vi "Kalibrierdaten.vi"() -> ()   [LabVIEW 2020, in "ABB-EL3000.lvlib" / "Allgemeine VI.lvlib"]
uses:
  Allgemeine VI.lvlib
  Visualisierungs Elemente/Button.ctl
  Visualisierungs Elemente/Zahlen-Ausgabefeld.ctl
  Visualisierungs Elemente/Zahlen-Eingabefeld.ctl
  Auto Kalibrieren/Aktionen FGV AutoKAL Daten.ctl
  FGV Uras26 Aktion.ctl
  CAL-Daten Toleranz.ctl
  Aktionen Cal Daten speichern.ctl
  PMA/Kalibrieren/Kalibrieren.lvlib
  Allgemein/allgemeine Sub-VIs.lvlib
  Auto Kalibrieren/Auto Kalibrieren.lvlib
  FID/FID Kalibrierung/FID Kalibrierung.lvlib
panel:
  out "THC End 3":T1 format="%.4f"
  out "THC End 2":T1 format="%.4f"
  in  "O2 Zeit-E":T2 format="%#_5g"
  in  "O2 Zeit-0":T2 format="%#_5g"
  in  "O2 0-Grund.":T2 format="%#_5g"
  in  "O2 0-KAL":T2 format="%#_5g"
  in  "O2 E-Grund.":T2 format="%#_5g"
  in  "O2 E-KAL":T2 format="%#_5g"
  out "O2 Null":T1 format="%.4f"
  out "O2 End":T1 format="%.4f"
  in  "THC Zeit-E":T2 format="%#_5g"
  in  "THC Zeit-0":T2 format="%#_5g"
  in  "THC 0-Grund.":T2 format="%#_5g"
  in  "THC 0-KAL":T2 format="%#_5g"
  out "THC Null":T1 format="%.4f"
  in  "THC E-Grund.":T2 format="%#_5g"
  in  "THC E-KAL":T2 format="%#_5g"
  out "THC End1":T1 format="%.4f"
  in  "CO2 hi Zeit-E":T2 format="%#_5g"
  in  "CO2 hi 0-Grund.":T2 format="%#_5g"
  in  "CO2 hi 0-KAL":T2 format="%#_5g"
  in  "CO2 hi E-Grund.":T2 format="%#_5g"
  in  "CO2 hi E-KAL":T2 format="%#_5g"
  out "CO2 hi Null":T1 format="%.4f"
  out "CO2 hi End1":T1 format="%.4f"
  in  "CO2 hi Zeit-0":T2 format="%#_5g"
  in  "CO2 lo Zeit-E":T2 format="%#_5g"
  in  "CO2 lo 0-Grund.":T2 format="%#_5g"
  in  "CO2 lo 0-KAL":T2 format="%#_5g"
  out "CO2 lo Null":T1 format="%.4f"
  in  "CO2 lo E-Grund.":T2 format="%#_5g"
  in  "CO2 lo E-KAL":T2 format="%#_5g"
  out "CO2 lo End2":T1 format="%.4f"
  out "CO2 lo End1":T1 format="%.4f"
  in  "CO2 lo Zeit-0":T2 format="%#_5g"
  in  "CH4 Zeit-E":T2 format="%#_5g"
  in  "CH4 Zeit-0":T2 format="%#_5g"
  in  "CH4 0-Grund.":T2 format="%#_5g"
  in  "CH4 0-KAL":T2 format="%#_5g"
  in  "CH4 E-Grund.":T2 format="%#_5g"
  in  "CH4 E-KAL":T2 format="%#_5g"
  out "CH4 Null":T1 format="%.4f"
  out "CH4 End1":T1 format="%.4f"
  in  "CO lo Zeit-E":T2 format="%#_5g"
  in  "CO lo Zeit-0":T2 format="%#_5g"
  in  "CO lo 0-Grund.":T2 format="%#_5g"
  in  "CO lo 0-KAL":T2 format="%#_5g"
  out "CO lo Null":T1 format="%.4f"
  out "CO lo End3":T1 format="%.4f"
  in  "CO lo E-Grund.":T2 format="%#_5g"
  in  "CO lo E-KAL":T2 format="%#_5g"
  out "CO lo End2":T1 format="%.4f"
  out "CO lo End1":T1 format="%.4f"
  in  "speichern":T3
  in  "ABBRECHEN":T3
  # "0-Punkt"
  # "End-Punkt"
  # "0-Punkt Toleranz [abs]"
  # "End-Punkt Toleranz [%]"
  # "Aufschaltzeit Auto-KAL [sec]"
  # "letzte\nKalibrierung"
  # "Grund-\nkalibrierung"
  # "letzte\nKalibrierung"
  # "Grund-\nkalibrierung"
  # "0-Punkt"
  # "End-Punkt"
  # "MB 1"
  # "MB 2"
  # "MB 3"
  # "THC:"
  # "O2:"
  # "reserve:"
  # "CO2 lo:"
  # "CH4:"
  # "CO lo:"
  # "Kalibrierdaten"
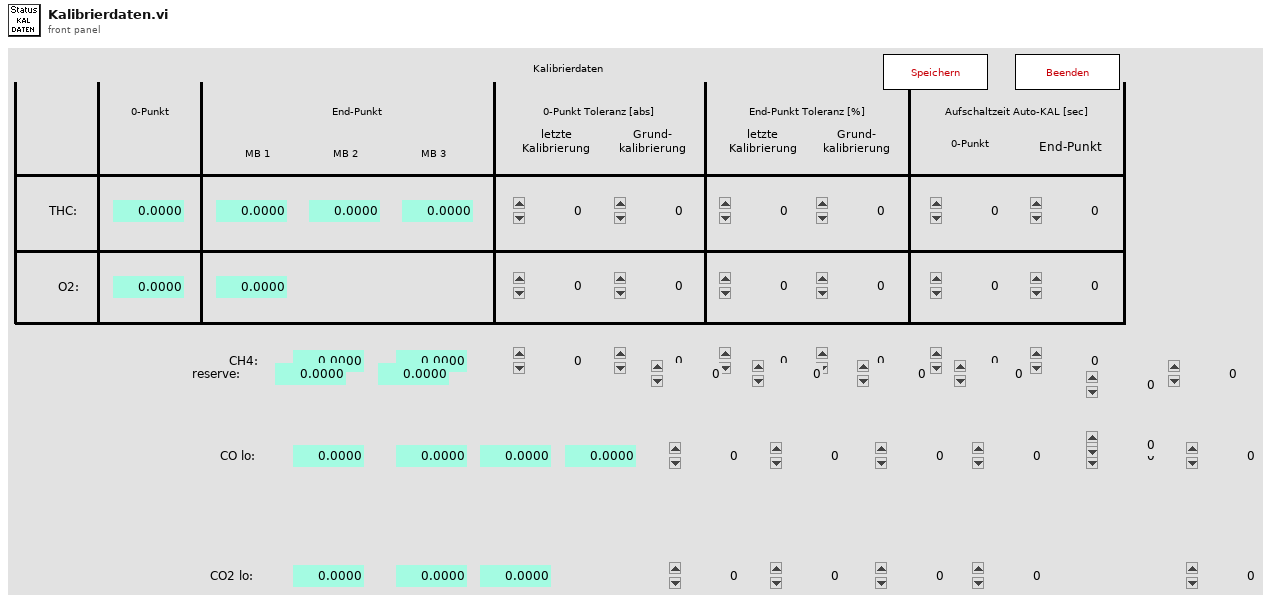
[diagram p1: front panel]
types:
  T1 = typedef "Zahlen-Ausgabefeld.ctl" = sgl
  T2 = typedef "Zahlen-Eingabefeld.ctl" = sgl
  T3 = typedef "Button.ctl" = bool
  T4 = typedef "ABB-EL3000.lvlib/Allgemeine VI.lvlib/FGV Uras26 Aktion.ctl" = enum16{"lesen", "CAL-Daten laden", "Messen", "Kalibrieren vorbereiten", "Kalibrieren", "CAL-Daten speichern", "Toleranz schreiben", "CAL-Daten kopieren"}
  T5 = typedef "Auto Kalibrieren.lvlib/Aktionen FGV AutoKAL Daten.ctl" = enum16{"lesen", "laden", "speichern", "Aufschaltzeit"}
  T6 = typedef "ABB-EL3000.lvlib/Allgemeine VI.lvlib/CAL-Daten Toleranz.ctl" = cluster{"CO lo 0-KAL":sgl, "CO lo 0-Grund":sgl, "CO lo E-KAL":sgl, "CO lo E-Grund":sgl, "CO hi 0-KAL":sgl, "CO hi 0-Grund":sgl, "CO hi E-KAL":sgl, "CO hi E-Grund":sgl, "CH4 0-KAL":sgl, "CH4 0-Grund":sgl, "CH4 E-KAL":sgl, "CH4 E-Grund":sgl, "THC 0-KAL":sgl, "THC 0-Grund":sgl, "THC E-KAL":sgl, "THC E-Grund":sgl, "NMHC 0-KAL":sgl, "NMHC 0-Grund":sgl, "NMHC E-KAL":sgl, "NMHC E-Grund":sgl, "O2 0-KAL":sgl, "O2 0-Grund":sgl, "O2 E-KAL":sgl, "O2 E-Grund":sgl}
  T7 = typedef "Auto Kalibrieren.lvlib/Auschaltzeiten Null Endpunktgase.ctl" = cluster{"CO lo 0":sgl, "CO lo E":sgl, "CO hi 0":sgl, "CO hi E":sgl, "CO2 lo 0":sgl, "CO2 lo E":sgl, "CH4 0":sgl, "CH4 E":sgl, "THC 0":sgl, "THC E":sgl, "O2 0":sgl, "O2 E":sgl}
  T8 = typedef "ABB-EL3000.lvlib/Allgemeine VI.lvlib/Aktionen Cal Daten speichern.ctl" = enum16{"Cal Daten", "Toleranzen", "PMA", "FID", "Cal Daten PMA", "Cal Daten FID"}
  T9 = typedef "ABB-EL3000.lvlib/Allgemeine VI.lvlib/CAL-Daten PMA.ctl" = cluster{"O2 Null":sgl, "O2 Steil":sgl[]}
  T10 = typedef "ABB-EL3000.lvlib/Allgemeine VI.lvlib/CAL-Daten FID.ctl" = cluster{"CH4 Null":sgl, "CH4 Steil":sgl[], "THC Null":sgl, "THC Steil":sgl[], "NMHC Null":sgl, "NMHC Steil":sgl[]}
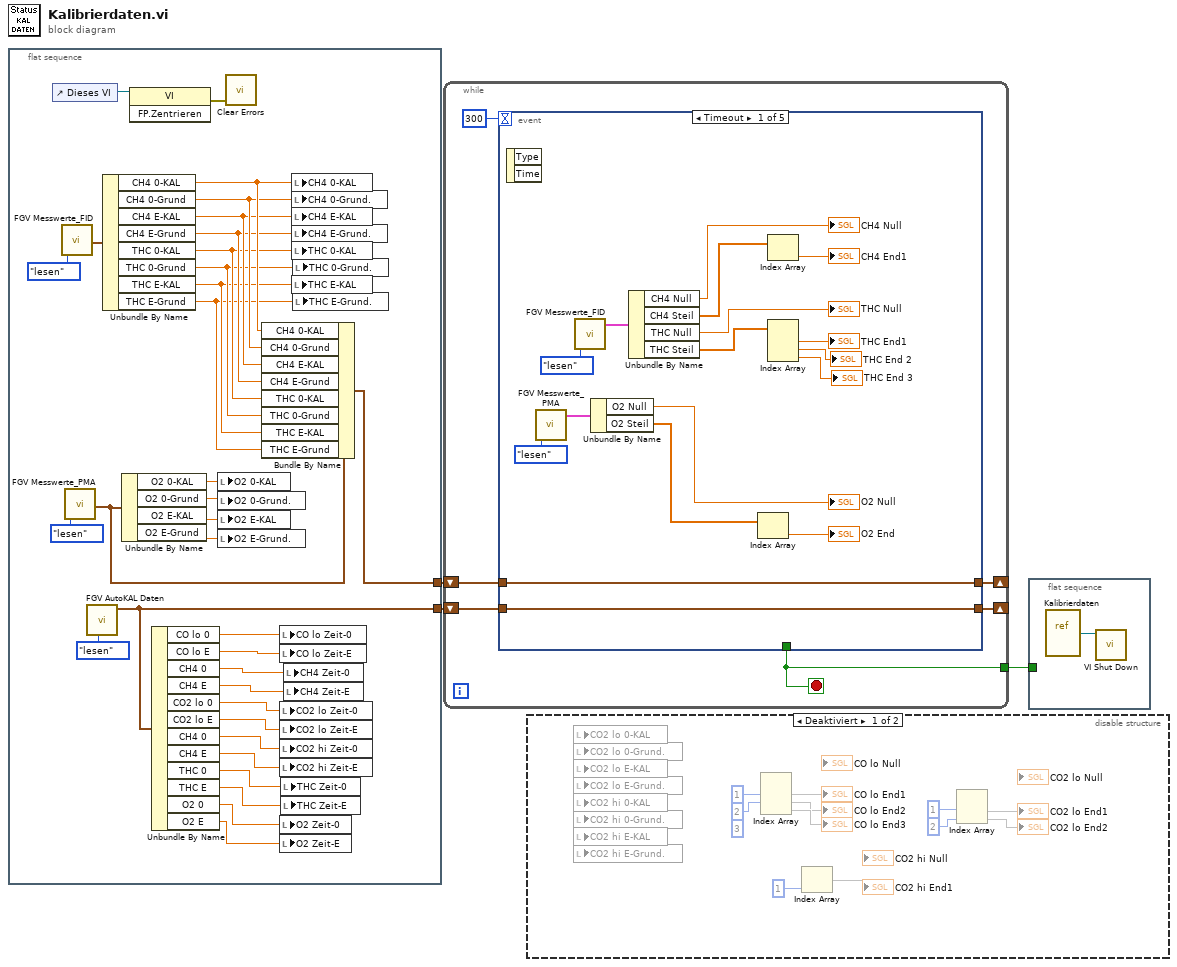
[diagram p0: block diagram]
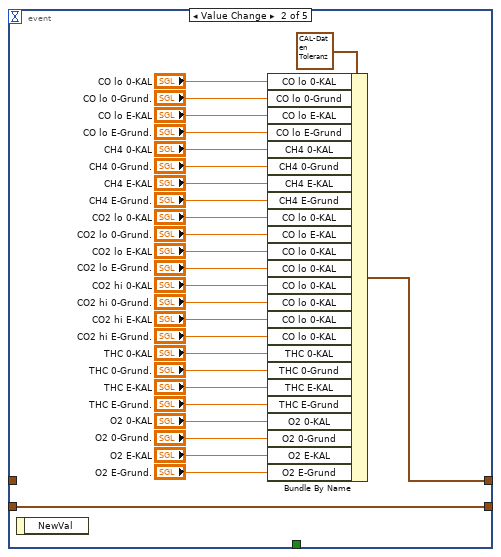
[diagram p3: hidden frame]
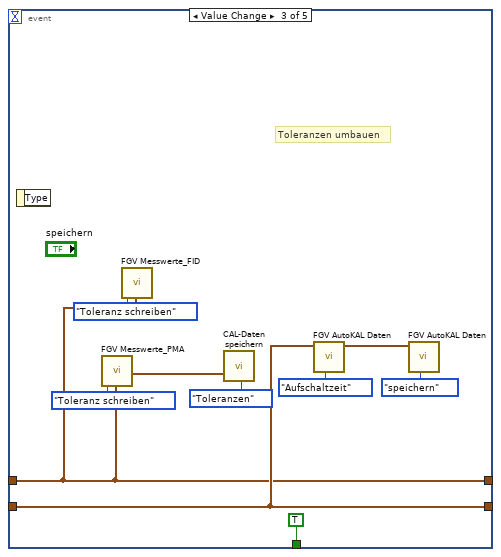
[diagram p4: hidden frame]
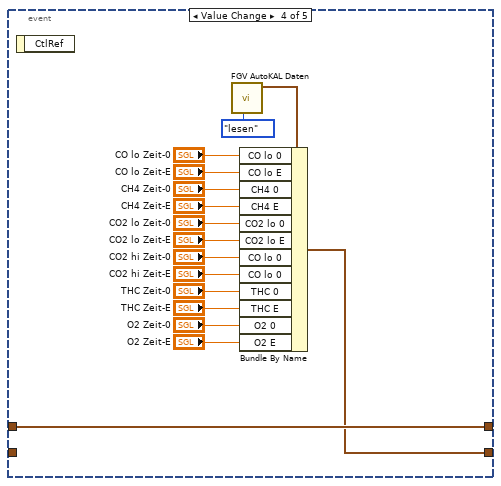
[diagram p5: hidden frame]
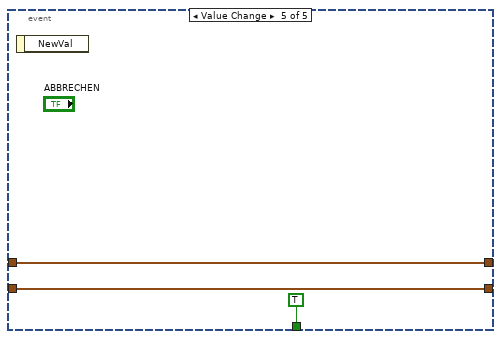
[diagram p6: hidden frame]
diagram:
  n1 = flat-sequence {
    tunnel: [w12] -> w2
    tunnel: [w33] -> w1
    frame #0 {
      n2 = control-ref of="Dieses VI"() -> (w16:refnum<vi>)
      n3 = call "FGV Messwerte_FID.vi"("Aktion"=FGV_Uras26_Aktion."lesen") -> ("CAL-Daten Tolernaz"=w13:T6)  [unwired: 19 in, 7 out]
      n4 = call "FGV Messwerte_PMA.vi"("Aktion"=FGV_Uras26_Aktion."lesen") -> ("CAL-Daten Tolernaz"=w35:T6)  [unwired: 19 in, 7 out]
      n5 = call "FGV AutoKAL Daten.vi"("Aktionen"=Aktionen_FGV_AutoKAL_Daten."lesen") -> ("Aufschaltzeiten"=w33:T7)  [unwired: 10 in]
      n6 = Unbundle By Name(w13) -> ("CH4 0-KAL"=w11:sgl, "CH4 0-Grund"=w10:sgl, "CH4 E-KAL"=w9:sgl, "CH4 E-Grund"=w8:sgl, "THC 0-KAL"=w7:sgl, "THC 0-Grund"=w6:sgl, "THC E-KAL"=w5:sgl, "THC E-Grund"=w4:sgl)
      n7 = Unbundle By Name(w35) -> ("O2 0-KAL"=w20:sgl, "O2 0-Grund"=w19:sgl, "O2 E-KAL"=w18:sgl, "O2 E-Grund"=w17:sgl)
      n8 = invoke class="VI" method="FP.Zentrieren"(reference=w16) -> (error out=w15:errorcluster)  [unwired: 2 in, 2 out]
      n9 = Unbundle By Name(w33) -> ("CO lo 0"=w31:sgl, "CO lo E"=w23:sgl, "CH4 0"=w24:sgl, "CH4 E"=w25:sgl, "CO2 lo 0"=w26:sgl, "CO2 lo E"=w27:sgl, "CH4 0"=w28:sgl, "CH4 E"=w29:sgl, "THC 0"=w30:sgl, "THC E"=w32:sgl, "O2 0"=w22:sgl, "O2 E"=w21:sgl)
      n10 = local write "O2 0-KAL"(w20) -> ()
      n11 = local write "O2 0-Grund."(w19) -> ()
      n12 = local write "O2 E-KAL"(w18) -> ()
      n13 = local write "O2 E-Grund."(w17) -> ()
      n14 = call <vilib>:"Clear Errors.vi"("error in (no error)"=w15) -> ()  [unwired: 5 in, 2 out]
      n15 = Bundle By Name(cluster=w35, "CH4 0-KAL"=w11, "CH4 0-Grund"=w10, "CH4 E-KAL"=w9, "CH4 E-Grund"=w8, "THC 0-KAL"=w7, "THC 0-Grund"=w6, "THC E-KAL"=w5, "THC E-Grund"=w4) -> (w12:T6)
      n16 = local write "CO lo Zeit-0"(w31) -> ()
      n17 = local write "CO lo Zeit-E"(w23) -> ()
      n18 = local write "CO2 lo Zeit-0"(w26) -> ()
      n19 = local write "CO2 lo Zeit-E"(w27) -> ()
      n20 = local write "CO2 hi Zeit-0"(w28) -> ()
      n21 = local write "CO2 hi Zeit-E"(w29) -> ()
      n22 = local write "O2 Zeit-0"(w22) -> ()
      n23 = local write "O2 Zeit-E"(w21) -> ()
      n24 = local write "THC Zeit-0"(w30) -> ()
      n25 = local write "THC Zeit-E"(w32) -> ()
      n26 = local write "CH4 Zeit-0"(w24) -> ()
      n27 = local write "CH4 Zeit-E"(w25) -> ()
      n28 = local write "CH4 0-KAL"(w11) -> ()
      n29 = local write "CH4 0-Grund."(w10) -> ()
      n30 = local write "CH4 E-KAL"(w9) -> ()
      n31 = local write "CH4 E-Grund."(w8) -> ()
      n32 = local write "THC 0-KAL"(w7) -> ()
      n33 = local write "THC E-KAL"(w5) -> ()
      n34 = local write "THC 0-Grund."(w6) -> ()
      n35 = local write "THC E-Grund."(w4) -> ()
    }
  }
  n36 = while {
    tunnel: [w41] -> w3
    shift-right: [w40] -> _
    shift-left: w2 -> [w39]
    shift-right: [w37] -> _
    shift-left: w1 -> [w38]
    stop <- w41 stop-if-true
    n37 = event shown="[0] Timeout" {
      selector: _ -> [_ _ _ _ _]
      dyn-events: _ -> [_ _ _ _ _]
      timeout: 300 -> [_ _ _ _ _]
      tunnel: [_ _ TRUE ("ABBRECHEN") _ TRUE ("ABBRECHEN")] -> w41
      tunnel: [w55 w65 w87 w112 w114] -> w40
      tunnel: w39 -> [w55 _ w87 w112 w114]
      tunnel: w38 -> [w54 w64 w91 _ w113]
      tunnel: [w54 w64 w91 w99 w113] -> w37
      event Timeout {
        n38 = event-data() -> ()  [unwired: 1 in, 2 out]
        n39 = call "FGV Messwerte_PMA.vi"("Aktion"=FGV_Uras26_Aktion."lesen") -> ("CAL-Daten"=w58:T9)  [unwired: 19 in, 7 out]
        n40 = call "FGV Messwerte_FID.vi"("Aktion"=FGV_Uras26_Aktion."lesen") -> ("CAL-Daten"=w49:T10)  [unwired: 19 in, 7 out]
        n41 = Unbundle By Name(w58) -> ("O2 Null"=→"O2 Null":sgl, "O2 Steil"=w52:sgl[])
        n42 = Unbundle By Name(w49) -> ("CH4 Null"=→"CH4 Null":sgl, "CH4 Steil"=w47:sgl[], "THC Null"=→"THC Null":sgl, "THC Steil"=w45:sgl[])
        n43 = Index Array(array=w52) -> (element=→"O2 End":sgl)  [unwired: 1 in]
        n44 = Index Array(array=w47) -> (element=→"CH4 End1":sgl)  [unwired: 1 in]
        n45 = Index Array(array=w45) -> (element #1=→"THC End1":sgl, element #2=→"THC End 2":sgl, element #3=→"THC End 3":sgl)  [unwired: 3 in]
      }
      event Value Change {
        n46 = event-data() -> ()  [unwired: 1 in, 1 out]
        n47 = Bundle By Name(cluster=T6 {"CO lo 0-KAL"=0.0, "CO lo 0-Grund"=0.0, "CO lo E-KAL"=0.0, "CO lo E-Grund"=0.0, "CO hi 0-KAL"=0.0, "CO hi 0-Grund"=0.0, "CO hi E-KAL"=0.0, "CO hi E-Grund"=0.0, "CH4 0-KAL"=0.0, "CH4 0-Grund"=0.0, "CH4 E-KAL"=0.0, "CH4 E-Grund"=0.0, "THC 0-KAL"=0.0, "THC 0-Grund"=0.0, "THC E-KAL"=0.0, "THC E-Grund"=0.0, "NMHC 0-KAL"=0.0, "NMHC 0-Grund"=0.0, "NMHC E-KAL"=0.0, "NMHC E-Grund"=0.0, "O2 0-KAL"=0.0, "O2 0-Grund"=0.0, "O2 E-KAL"=0.0, "O2 E-Grund"=0.0} ("CAL-Daten Tolernaz"), "CO lo 0-KAL"="CO lo 0-KAL", "CO lo 0-Grund"="CO lo 0-Grund.", "CO lo E-KAL"="CO lo E-KAL", "CO lo E-Grund"="CO lo E-Grund.", "CH4 0-KAL"="CH4 0-KAL", "CH4 0-Grund"="CH4 0-Grund.", "CH4 E-KAL"="CH4 E-KAL", "CH4 E-Grund"="CH4 E-Grund.", "CO lo 0-KAL"="CO2 lo 0-KAL", "CO lo E-KAL"="CO2 lo 0-Grund.", "CO lo 0-KAL"="CO2 lo E-KAL", "CO lo 0-KAL"="CO2 lo E-Grund.", "CO lo 0-KAL"="CO2 hi 0-KAL", "CO lo 0-KAL"="CO2 hi 0-Grund.", "CO lo 0-KAL"="CO2 hi E-KAL", "CO lo 0-KAL"="CO2 hi E-Grund.", "THC 0-KAL"="THC 0-KAL", "THC 0-Grund"="THC 0-Grund.", "THC E-KAL"="THC E-KAL", "THC E-Grund"="THC E-Grund.", "O2 0-KAL"="O2 0-KAL", "O2 0-Grund"="O2 0-Grund.", "O2 E-KAL"="O2 E-KAL", "O2 E-Grund"="O2 E-Grund.") -> (w65:T6)
      }
      event Value Change {
        # "Toleranzen umbauen"
        n48 = event-data() -> ()  [unwired: 1 in, 1 out]
        n49 = call "FGV Messwerte_PMA.vi"("Aktion"=FGV_Uras26_Aktion."Toleranz schreiben", "CAL-Daten Tolernaz"=w87) -> ("CAL-Daten Tolernaz"=w93:T6)  [unwired: 18 in, 7 out]
        n50 = call "FGV Messwerte_FID.vi"("Aktion"=FGV_Uras26_Aktion."Toleranz schreiben", "CAL-Daten Tolernaz"=w87) -> ()  [unwired: 18 in, 8 out]
        n51 = call "CAL-Daten speichern.vi"("CAL-Daten Tolernaz"=w93, "Aktionen Kal Daten speichern"=Aktionen_Cal_Daten_speichern."Toleranzen") -> ()  [unwired: 18 in]
        n52 = call "FGV AutoKAL Daten.vi"("Aktionen"=Aktionen_FGV_AutoKAL_Daten."Aufschaltzeit", "Aufschaltzeiten"=w91) -> ("Aufschaltzeiten"=w89:T7)  [unwired: 9 in]
        n53 = call "FGV AutoKAL Daten.vi"("Aktionen"=Aktionen_FGV_AutoKAL_Daten."speichern", "Aufschaltzeiten"=w89) -> ()  [unwired: 9 in, 1 out]
      }
      event Value Change {
        n54 = event-data() -> ()  [unwired: 1 in, 1 out]
        n55 = call "FGV AutoKAL Daten.vi"("Aktionen"=Aktionen_FGV_AutoKAL_Daten."lesen") -> ("Aufschaltzeiten"=w110:T7)  [unwired: 10 in]
        n56 = Bundle By Name(cluster=w110, "CO lo 0"="CO lo Zeit-0", "CO lo E"="CO lo Zeit-E", "CH4 0"="CH4 Zeit-0", "CH4 E"="CH4 Zeit-E", "CO2 lo 0"="CO2 lo Zeit-0", "CO2 lo E"="CO2 lo Zeit-E", "CO lo 0"="CO2 hi Zeit-0", "CO lo 0"="CO2 hi Zeit-E", "THC 0"="THC Zeit-0", "THC E"="THC Zeit-E", "O2 0"="O2 Zeit-0", "O2 E"="O2 Zeit-E") -> (w99:T7)
      }
      event Value Change {
        n57 = event-data() -> ()  [unwired: 1 in, 1 out]
      }
    }
  }
  n58 = disable-structure shown="Deaktiviert" {
    frame Disabled {
      (unwired) 3 ("Index")
      n59 = local read "CO2 lo 0-KAL"() -> ()  [unwired: 1 in]
      n60 = local read "CO2 lo 0-Grund."() -> ()  [unwired: 1 in]
      n61 = local read "CO2 lo E-KAL"() -> ()  [unwired: 1 in]
      n62 = local read "CO2 lo E-Grund."() -> ()  [unwired: 1 in]
      n63 = local read "CO2 hi 0-KAL"() -> ()  [unwired: 1 in]
      n64 = local read "CO2 hi 0-Grund."() -> ()  [unwired: 1 in]
      n65 = local read "CO2 hi E-KAL"() -> ()  [unwired: 1 in]
      n66 = local read "CO2 hi E-Grund."() -> ()  [unwired: 1 in]
      n67 = Index Array(index #1=1 ("Index"), index #2=2 ("Index")) -> (element #1=→"CO lo End1", element #2=→"CO lo End2", element #3=→"CO lo End3")  [unwired: 2 in]
      n68 = Index Array(index=1 ("Index")) -> (element=→"CO2 hi End1")  [unwired: 1 in]
      n69 = Index Array(index #1=1 ("Index"), index #2=2 ("Index")) -> (element #1=→"CO2 lo End1", element #2=→"CO2 lo End2")  [unwired: 1 in]
    }
    frame Enabled {
    }
  }
  n70 = flat-sequence {
    tunnel: w3 -> [_]
    frame #0 {
      n71 = vi-ref "Kalibrierdaten.vi"() -> (w127:refnum<vi>)
      n72 = call "VI Shut Down.vi"("VI Referenz"=w127) -> ()  [unwired: 11 in]
    }
  }
